vi "Filter.vi"() -> ()   [LabVIEW 2011]
doc: "This example shows some results of the use of the Filter Express VI.\n\nThis example uses the following Express VIs: Simulate Signal, Filter, Spectral Measurements, Tone Measurements, and Build XY Graph."
uses:
  Instance           1 14Saved   Filter .vi
  Instance           2 14Saved   Filter .vi
  Instance           5 14Saved   Filter .vi
  Instance           4 14Saved   Filter .vi
  Instance           3 14Saved   Filter .vi
  Instance           8 14Saved   Filter .vi
  Instance           7 14Saved   Filter .vi
  <vilib>/express/express analysis/Spectral/Block/exnSpectralBlock spectral measurements peak poly.vi
  <vilib>/express/express analysis/Spectral/Block/exnSpectralBlock spectral measurements peak DDT.vi
  <vilib>/express/express analysis/Spectral/XNode/ExpressSpectralMeasurementsBlockNode.xnode
panel:
  out "Single Tone Results":cluster{"Y":dbl[], "Y":dbl[]}[](graph)=[{"Y"=[489.00000000005195], "Y"=[1.9989155027865388]}, {"Y"=[489.00000000011886], "Y"=[0.0020146632305762225]}, {"Y"=[489.000000000171], "Y"=[0.0002518384154478026]}]
  out "FFT Results (Lin)":dynamicdata(graph)=[{"t0"=timestamp(0 s since 1904-01-01), "dt"=10.0, "Y"=array[1000 elements], "attributes"=variant("NI_ChannelName"=variant(string "Sine (FFT - (Peak))"), "NI_ExpIsRelativeTime"=variant(bool TRUE), "NI_ExpStartTimeStamp"=variant(timestamp timestamp(3198709062.64 s since 1904-01-01)), "NI_ExpTimeStamp"=variant(timestamp timestamp(3198709138.44 s since 1904-01-01)), "NI_ExpXDimension"=variant(string "f"), "NI_OriginalChannelName"=variant(string "Sine"))}, {"t0"=timestamp(0 s since 1904-01-01), "dt"=10.0, "Y"=array[1000 elements], "attributes"=variant("NI_ChannelName"=variant(string "Sine (FFT - (Peak))"), "NI_ExpIsRelativeTime"=variant(bool TRUE), "NI_ExpStartTimeStamp"=variant(timestamp timestamp(3198709062.64 s since 1904-01-01)), "NI_ExpTimeStamp"=variant(timestamp timestamp(3198709138.44 s since 1904-01-01)), "NI_ExpXDimension"=variant(string "f"), "NI_OriginalChannelName"=variant(string "Sine"))}, {"t0"=timestamp(0 s since 1904-01-01), "dt"=10.0, "Y"=array[1000 elements], "attributes"=variant("NI_ChannelName"=variant(string "Sine (FFT - (Peak))"), "NI_ExpIsRelativeTime"=variant(bool TRUE), "NI_ExpStartTimeStamp"=variant(timestamp timestamp(3198709062.64 s since 1904-01-01)), "NI_ExpTimeStamp"=variant(timestamp timestamp(3198709138.44 s since 1904-01-01)), "NI_ExpXDimension"=variant(string "f"), "NI_OriginalChannelName"=variant(string "Sine"))}]
  out "FFT Results (Log)":dynamicdata(graph)=[{"t0"=timestamp(0 s since 1904-01-01), "dt"=10.0, "Y"=array[1000 elements], "attributes"=variant("NI_ChannelName"=variant(string "Sine (FFT - (Peak))"), "NI_ExpIsRelativeTime"=variant(bool TRUE), "NI_ExpStartTimeStamp"=variant(timestamp timestamp(3198709062.64 s since 1904-01-01)), "NI_ExpTimeStamp"=variant(timestamp timestamp(3198709138.44 s since 1904-01-01)), "NI_ExpXDimension"=variant(string "f"), "NI_OriginalChannelName"=variant(string "Sine"))}, {"t0"=timestamp(0 s since 1904-01-01), "dt"=10.0, "Y"=array[1000 elements], "attributes"=variant("NI_ChannelName"=variant(string "Sine (FFT - (Peak))"), "NI_ExpIsRelativeTime"=variant(bool TRUE), "NI_ExpStartTimeStamp"=variant(timestamp timestamp(3198709062.64 s since 1904-01-01)), "NI_ExpTimeStamp"=variant(timestamp timestamp(3198709138.44 s since 1904-01-01)), "NI_ExpXDimension"=variant(string "f"), "NI_OriginalChannelName"=variant(string "Sine"))}, {"t0"=timestamp(0 s since 1904-01-01), "dt"=10.0, "Y"=array[1000 elements], "attributes"=variant("NI_ChannelName"=variant(string "Sine (FFT - (Peak))"), "NI_ExpIsRelativeTime"=variant(bool TRUE), "NI_ExpStartTimeStamp"=variant(timestamp timestamp(3198709062.64 s since 1904-01-01)), "NI_ExpTimeStamp"=variant(timestamp timestamp(3198709138.44 s since 1904-01-01)), "NI_ExpXDimension"=variant(string "f"), "NI_OriginalChannelName"=variant(string "Sine"))}]
  in  "Frequency":dbl(slide)=489.0 min=1.0 max=5000.0 step=1.0 scale=1.0..5000.0
  out "Signal":dynamicdata(graph)=[{"t0"=timestamp(75.8 s since 1904-01-01), "dt"=5e-05, "Y"=array[2000 elements], "attributes"=variant("NI_ChannelName"=variant(string "Sine (Filtered)"), "NI_ExpIsRelativeTime"=variant(bool TRUE), "NI_ExpStartTimeStamp"=variant(timestamp timestamp(3198709062.64 s since 1904-01-01)), "NI_ExpTimeStamp"=variant(timestamp timestamp(3198709138.44 s since 1904-01-01)), "NI_ExpXDimension"=variant(string "t"), "NI_OriginalChannelName"=variant(string "Sine"))}, {"t0"=timestamp(75.8 s since 1904-01-01), "dt"=5e-05, "Y"=array[2000 elements], "attributes"=variant("NI_ChannelName"=variant(string "Sine (Filtered)"), "NI_ExpIsRelativeTime"=variant(bool TRUE), "NI_ExpStartTimeStamp"=variant(timestamp timestamp(3198709062.64 s since 1904-01-01)), "NI_ExpTimeStamp"=variant(timestamp timestamp(3198709138.44 s since 1904-01-01)), "NI_ExpXDimension"=variant(string "t"), "NI_OriginalChannelName"=variant(string "Sine"))}, {"t0"=timestamp(75.8 s since 1904-01-01), "dt"=5e-05, "Y"=array[2000 elements], "attributes"=variant("NI_ChannelName"=variant(string "Sine (Filtered)"), "NI_ExpIsRelativeTime"=variant(bool TRUE), "NI_ExpStartTimeStamp"=variant(timestamp timestamp(3198709062.64 s since 1904-01-01)), "NI_ExpTimeStamp"=variant(timestamp timestamp(3198709138.44 s since 1904-01-01)), "NI_ExpXDimension"=variant(string "t"), "NI_OriginalChannelName"=variant(string "Sine"))}]
  in  "stop":bool
  # "This Example shows the results of filter functions."
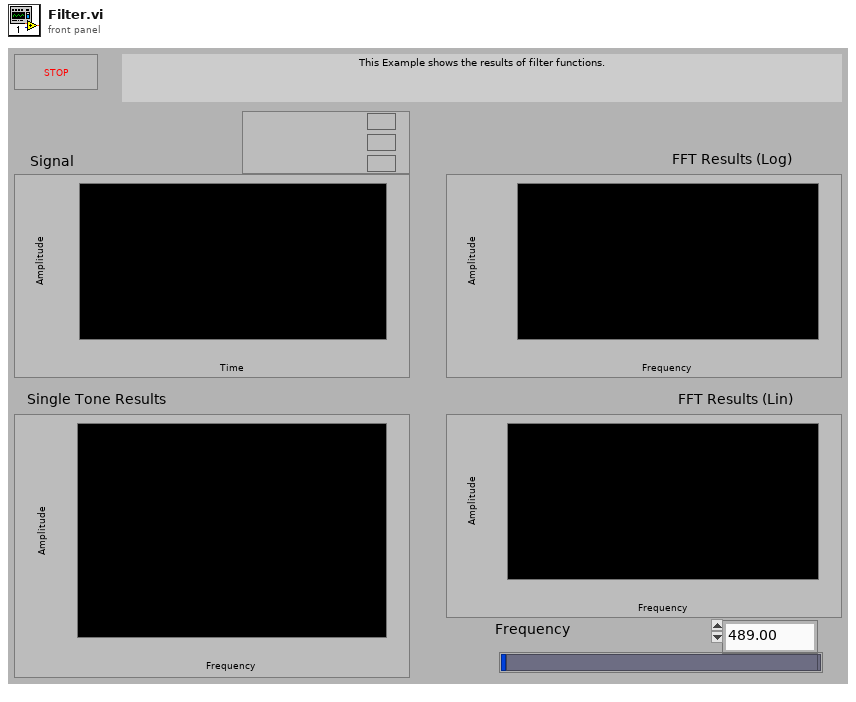
[diagram p1: front panel]
types:
  T1 = cluster{"averaging mode":u16, "weighting mode":u16, "number of averages":u32}
  T2 = cluster{"dB On (F)":bool, "unwrap phase (F)":bool, "convert to degree (F)":bool}
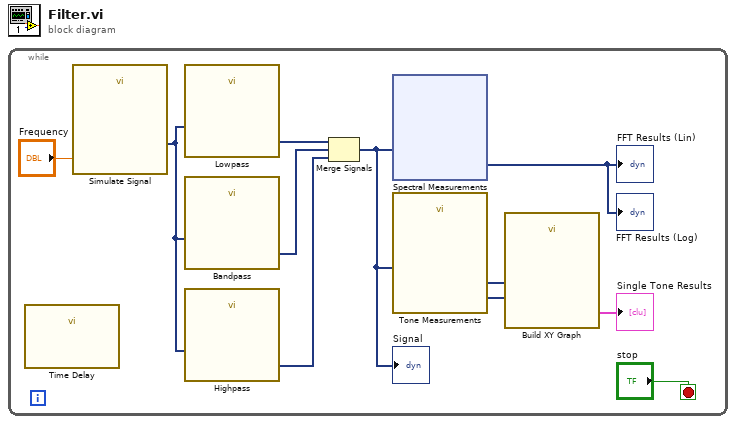
[diagram p0: block diagram]
diagram:
  n1 = while {
    stop <- "stop" stop-if-true
    n2 = call "Time Delay"() -> ()  [unwired: 11 in, 1 out]
    n3 = call "Simulate Signal"("Frequency"="Frequency") -> ("Sine"=w7:dynamicdata)  [unwired: 13 in, 1 out]
    n4 = call "Lowpass"("Signal"=w7) -> ("Filtered Signal"=w9:dynamicdata)  [unwired: 9 in, 1 out]
    n5 = call "Bandpass"("Signal"=w7) -> ("Filtered Signal"=w8:dynamicdata)  [unwired: 9 in, 1 out]
    n6 = call "Highpass"("Signal"=w7) -> ("Filtered Signal"=w6:dynamicdata)  [unwired: 9 in, 1 out]
    n7 = Merge Signals(w9, w8, w6) -> (w4:dynamicdata)
    "Signal" <- w4
    n8 = xnode "Spectral Measurements"("Signals"=w4) -> ("FFT - (Peak)"=→"FFT Results (Log)" →"FFT Results (Lin)":dynamicdata)  [unwired: 1 in, 2 out]
    n9 = call "Tone Measurements"("Signals"=w4) -> ("Frequency"=w3:dynamicdata, "Amplitude"=w2:dynamicdata)  [unwired: 8 in, 1 out]
    n10 = call "Build XY Graph"("Y Input"=w2, "X Input"=w3) -> ("XY Graph"=→"Single Tone Results":cluster{"Y":dbl[], "Y":dbl[]}[])  [unwired: 8 in, 1 out]
  }
